vi "Day4.vi"(11 "Input":string="MMMSXXMASM\nMSAMXMSMSA\nAMXSXMAAMM\nMSAMASMSMX\nXMASAMXAMM\nXXAMMXXAMA\nSMSMSASXSS\nSAXAMASAAA\nMAMMMXMMMM\nMXMXAXMASX") -> (3 "Result":i64)   [LabVIEW 2024]
uses:
  Day4Direction.ctl
  <userlib>/_OpenG.lib/string/string.llb/openg_string.lvlib
panel:
  out "Array":i64[][](array[numeric])
  out "Character Array":string[][](array[string])
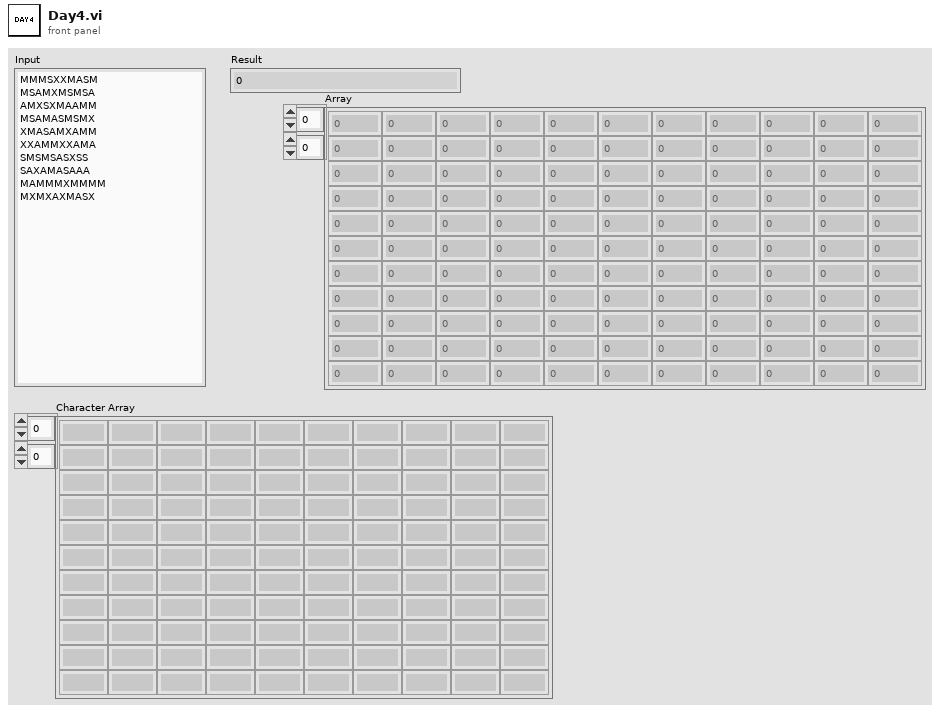
[diagram p1: front panel]
types:
  T1 = typedef "Day4Direction.ctl" = enum16{"BR", "BL", "B", "R", "L", "UR", "UL", "U"}
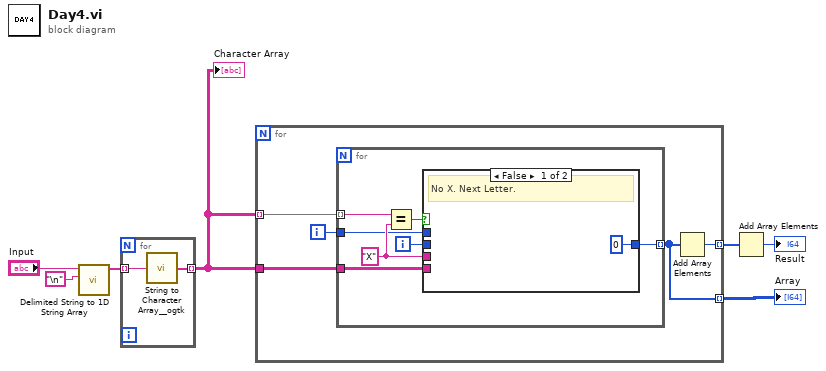
[diagram p0: block diagram]
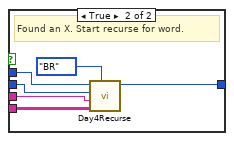
[diagram p2: hidden frame]
diagram:
  n1 = call <vilib>:"Delimited String to 1D String Array.vi"("delimiter"="\n", "delimited string"="Input") -> ("string array"=w5:string[])  [unwired: 9 in]
  n2 = for {
    tunnel: w5 -> [w9] mode=indexing
    tunnel: [w8] -> w1 mode=indexing
    n3 = call <userlib>:"String to Character Array__ogtk.vi"("Input String"=w9) -> ("Character Array"=w8:string[])
  }
  "Character Array" <- w1
  n4 = for {
    tunnel: w1 -> [w14] mode=indexing
    tunnel: w1 -> [w12]
    tunnel: [w11] -> w4 mode=indexing
    tunnel: [w10] -> w2 mode=indexing
    i -> [w13]
    n5 = for {
      tunnel: w14 -> [w21] mode=indexing
      tunnel: w13 -> [w18]
      tunnel: w12 -> [w17]
      tunnel: [w15] -> w10 mode=indexing
      i -> [w16]
      w19 = "X" ("y")
      n6 = Equal?(x=w21, y=w19) -> (x = y?=w20:bool)
      n7 = case shown="False" w20 {
        tunnel: w19 -> [_ w28]
        tunnel: w18 -> [_ w25]
        tunnel: w17 -> [_ w27]
        tunnel: w16 -> [_ w24]
        tunnel: [i64 0 ("XMASCount") w23] -> w15
        frame False {
          # "No X. Next Letter."
        }
        frame True {
          # "Found an X. Start recurse for word."
          n8 = call "Day4Recurse.vi"("Direction"=Day4Direction."BR", "Character Array"=w27, "Letter"=w28, "YIndex"=w24, "XIndex"=w25) -> ("XMASCount"=w23:i64)  [unwired: 6 in]
        }
      }
    }
    n9 = Add Array Elements(numeric array=w10) -> (sum=w11:i64)
  }
  "Array" <- w2
  n10 = Add Array Elements(numeric array=w4) -> (sum=→"Result":i64)
